vi "Get State ID.vi"(0 "SystemLink connection in":T1, 5 "state name":string, 11 "error in (no error)":errorcluster) -> (4 "SystemLink connection out":T1, 6 "state name out":string, 8 "state ID":string, 15 "error out":errorcluster)   [LabVIEW 2017, in "SystemLink_States_API.lvlib"]
doc: "Returns the State ID for the specified state name"
uses:
  SystemLink_States_API.lvlib
  systemlink connection.ctl
  <vilib>/httpClient/ClientHandle.ctl
  <vilib>/httpClient/LabVIEWHTTPClient.lvlib
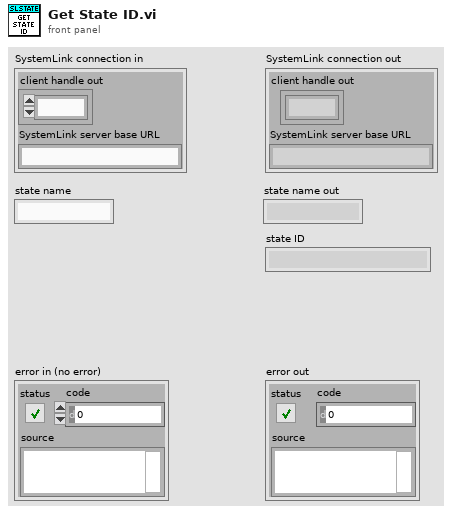
[diagram p1: front panel]
types:
  T1 = typedef "SystemLink_States_API.lvlib/systemlink connection.ctl" = cluster{"client handle out":T2, "SystemLink server base URL":string}
  T2 = typedef "LabVIEWHTTPClient.lvlib/ClientHandle.ctl" = refnum<k1>
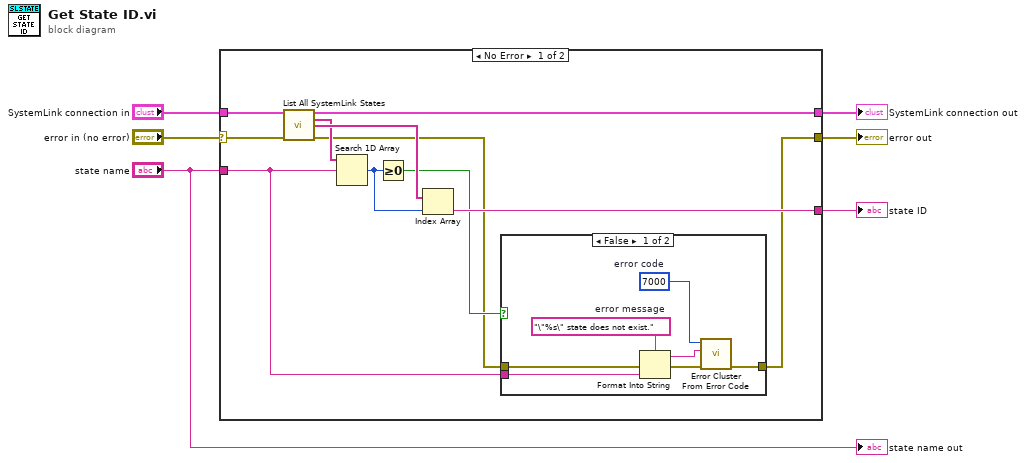
[diagram p0: block diagram]
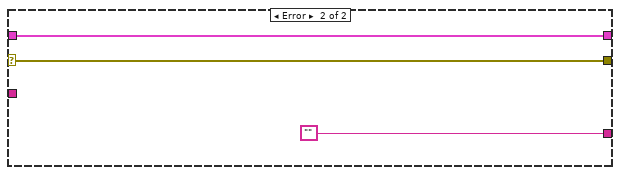
[diagram p3: hidden frame]
diagram:
  n1 = case shown="No Error" "error in (no error)" {
    selector: "error in (no error)" -> [w11 w28]
    tunnel: [w17 "" ("Data Type and Default Value")] -> w6
    tunnel: "state name" -> [w9 _]
    tunnel: [w13 w27] -> w5
    tunnel: "SystemLink connection in" -> [w12 w27]
    tunnel: [w7 w28] -> w3
    frame No Error {
      n2 = call "List All SystemLink States.vi"("SystemLink connection in"=w12, "error in (no error)"=w11) -> ("SystemLink connection out"=w13:T1, "SystemLink State Names"=w14:string[], "SystemLink State IDs"=w15:string[], "error out"=w8:errorcluster)  [unwired: 10 in]
      n3 = Search 1D Array(1D array=w14, element=w9) -> (index of element=w16:i32)  [unwired: 1 in]
      n4 = Greater Or Equal To 0?(x=w16) -> (x >= 0?=w10:bool)
      n5 = Index Array(array=w15, index=w16) -> (element=w17:string)
      n6 = case shown="False" w10 {
        tunnel: w8 -> [w20 w25]
        tunnel: w9 -> [w19 _]
        tunnel: [w18 w25] -> w7
        frame False {
          w23 = "\"%s\" state does not exist."  # error message
          w24 = 7000  # error code
          n7 = Format Into String(format string=w23, error in=w20, w19) -> (resulting string=w22:string, error out=w21:errorcluster)  [unwired: 1 in]
          n8 = call <vilib>:"Error Cluster From Error Code.vi"("error in (no error)"=w21, "error message (\"\")"=w22, "error code (0)"=w24) -> ("error out"=w18:errorcluster)  [unwired: 6 in]
        }
        frame True {
        }
      }
    }
    frame Error {
    }
  }
  "state ID" <- w6
  "SystemLink connection out" <- w5
  "error out" <- w3
  "state name out" <- "state name"
